vi "PropertyChangedEventCallbackForHistogram.vi"(4 "?":refnum<vi>, 5 "Event Data":cluster{"sender":refnum<k24>, "e":refnum<k24>}, 6 "Control Ref":refnum<k24>, 7 "Event Common Data":T1) -> ()   [LabVIEW 2019]
uses:
  D:/SDK/PMQI-LabViewSamples/Examples/Dependencies/PVCamNET.dll
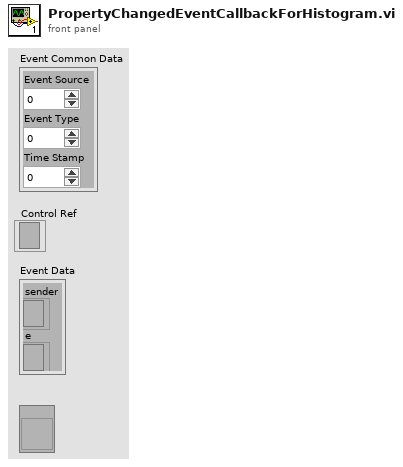
[diagram p1: front panel]
types:
  T1 = cluster{"Event Source":i32, "Event Type":u32, "Time Stamp":u32}
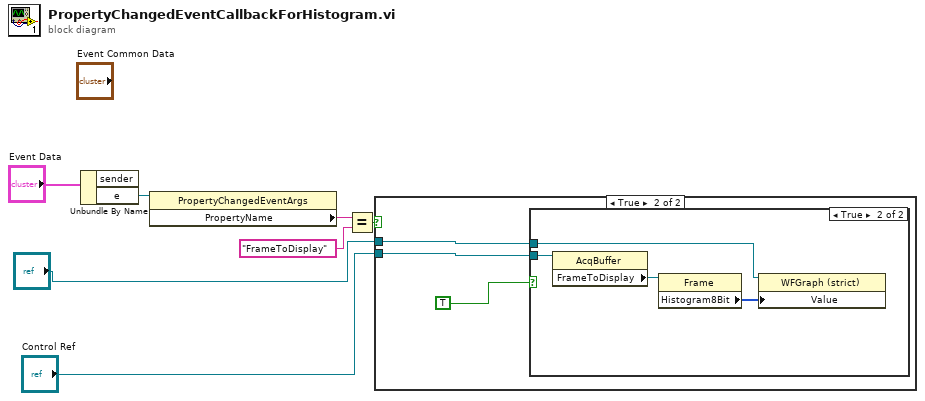
[diagram p0: block diagram]
diagram:
  n1 = Unbundle By Name("Event Data") -> ("e"=w7:refnum<k24>)  [unwired: 1 out]
  n2 = property class="PropertyChangedEventArgs"(reference=w7) -> ("PropertyName"=w6:string)  [unwired: 1 in, 2 out]
  n3 = Equal?(x=w6, y="FrameToDisplay") -> (x = y?=w4:bool)
  n4 = case shown="True" w4 {
    tunnel: "?" -> [_ w10]
    tunnel: "Control Ref" -> [_ w9]
    frame False {
    }
    frame True {
      n5 = case shown="True" TRUE {
        tunnel: w10 -> [_ w14]
        tunnel: w9 -> [_ w12]
        frame False {
        }
        frame True {
          n6 = property class="AcqBuffer"(reference=w12) -> ("FrameToDisplay"=w11:refnum<k24>)  [unwired: 1 in, 2 out]
          n7 = property class="Frame"(reference=w11) -> ("Histogram8Bit"=w13:u32[])  [unwired: 1 in, 2 out]
          n8 = property class="WFGraph (strict)"(reference=w14, "Value"=w13) -> ()  [unwired: 1 in, 2 out]
        }
      }
    }
  }
